vi "TitleBar.Start.vi"(5 "Autoshutdown? (T)":bool=TRUE, 8 "error in (no error)":errorcluster, 11 "NewTemplate in":refnum<class "TitleBar.lvclass">) -> (0 "error out":errorcluster, 1 "StartupHandshake out":refnum<class "RQMHStartup.lvclass">, 2 "TitleBar":cluster{"Broadcasts":T1, "Broadcasts":T2}, 3 "TitleBar":refnum<class "TitleBar.lvclass">)   [LabVIEW 2024, in "TitleBar.lvclass"]
uses:
  TitleBar.lvclass
  C:/Github/JQMH/JQMHCore/Module/RQMHModule.lvclass
  JQMHCore/Module/StandardBroadcasts.ctl
  JQMHCore/Shared/Died.ctl
  JQMHCore/Module/Started.ctl
  Broadcast Events--cluster.ctl
  Stopped.ctl
  Maximise.ctl
  JQMHCore/Module/RQMHModule.lvclass
  Minimise.ctl
  ClosePress.ctl
  JQMHCore/JQMHStartup/RQMHStartup.lvclass
  JQMHCore/Shared/RQMHShared.lvlib
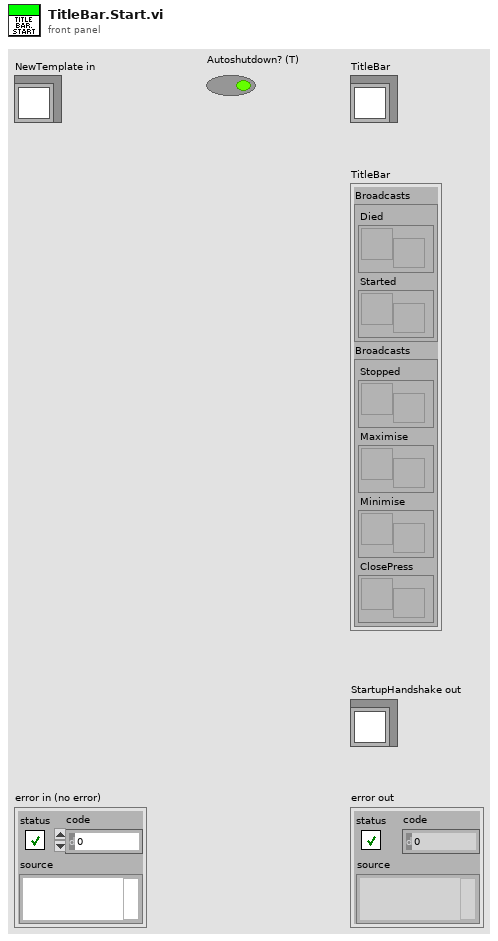
[diagram p1: front panel]
types:
  T1 = typedef "RQMHModule.lvclass/StandardBroadcasts.ctl" = cluster{"Died":refnum<user-event>, "Started":refnum<user-event>}
  T2 = typedef "TitleBar.lvclass/Broadcast Events--cluster.ctl" = cluster{"Stopped":refnum<user-event>, "Maximise":refnum<user-event>, "Minimise":refnum<user-event>, "ClosePress":refnum<user-event>}
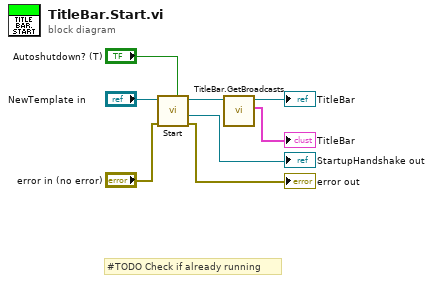
[diagram p0: block diagram]
diagram:
  # "#TODO Check if already running"
  n1 = call "Start.vi"("Autoshutdown? (T)"="Autoshutdown? (T)", "error in (no error)"="error in (no error)", "JQMHCore in"="NewTemplate in") -> ("error out"=→"error out":errorcluster, "StartupHandshake out"=→"StartupHandshake out":refnum<class "RQMHStartup.lvclass">, "JQMHCore out"=w4:refnum<class "TitleBar.lvclass">)  [unwired: 6 in]
  n2 = call "TitleBar.GetBroadcasts.vi"("NewTemplate in"=w4) -> ("TemplateModule"=→"TitleBar":cluster{"Broadcasts":T1, "Broadcasts":T2}, "NewTemplate out"=→"TitleBar":refnum<class "TitleBar.lvclass">)  [unwired: 9 in]
